vi "PingPongBRAMTop.vi"(5 "Memories":T3, 7 "ReverseLineRead?":bool, 8 "Input Valid":bool, 9 "Line Status In":T2, 11 "Data In":i16[](array[numeric])=[0, 0, 0, 0]) -> (0 "Output Valid":bool, 1 "Line Status Out":T2, 3 "Data Out":i16[](array[numeric]))   [LabVIEW 2014]
doc: "This VI ping pongs data between two Block RAM (memory)."
uses:
  Acquisition Engine/Acquisition Status.ctl
panel:
  # "Copyright 2014 Vidrio Technologies\nScanImage 5 software is licensed under the Apache License, Version 2.0 (the \"License\"); you may not use any files contained\nwithin the ScanImage 5 release except in compliance with the License. You may obtain a copy of the License at\n http://www.apache.org/licenses/LICENSE-2.0\nUnless required by applicable law or agreed to in writing, software distributed under the License is distributed on an\n\"AS IS\" BASIS, WITHOUT WARRANTIES OR CONDITIONS OF ANY KIND, either express or implied. See the License for the\n specific language governing permissions and limitations under the License."
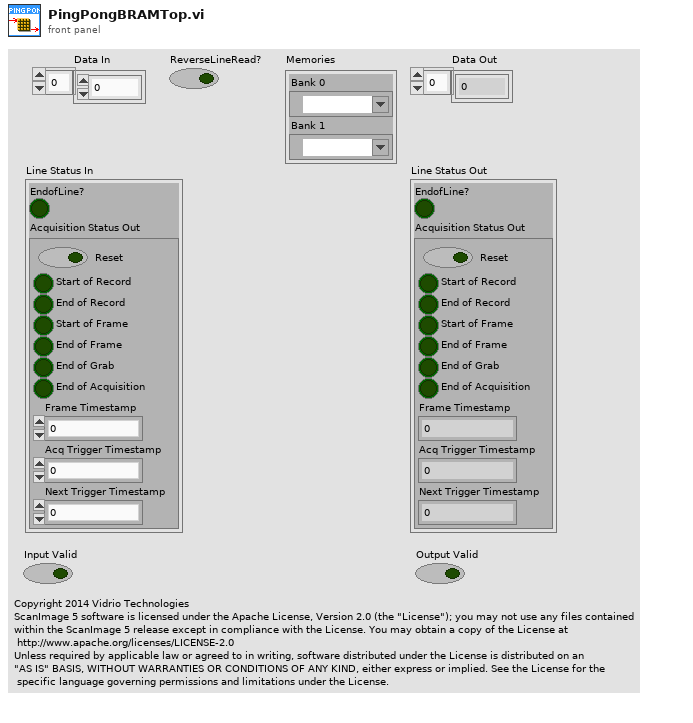
[diagram p1: front panel]
types:
  T1 = typedef "Acquisition Status.ctl" = cluster{"Reset":bool, "Start of Record":bool, "End of Record":bool, "Start of Frame":bool, "End of Frame":bool, "End of Grab":bool, "End of Acquisition":bool, "Frame Timestamp":u64, "Acq Trigger Timestamp":u64, "Next Trigger Timestamp":u64}
  T2 = cluster{"EndofLine?":bool, "Acquisition Status Out":T1}
  T3 = cluster{"Bank 0":refnum<k21>, "Bank 1":refnum<k21>}
  T4 = cluster{"Pixel Data":i16[], "Timestamps":cluster{"Frame Timestamp":u64, "Acq Trigger Timestamp":u64, "Next Trigger Timestamp":u64}}
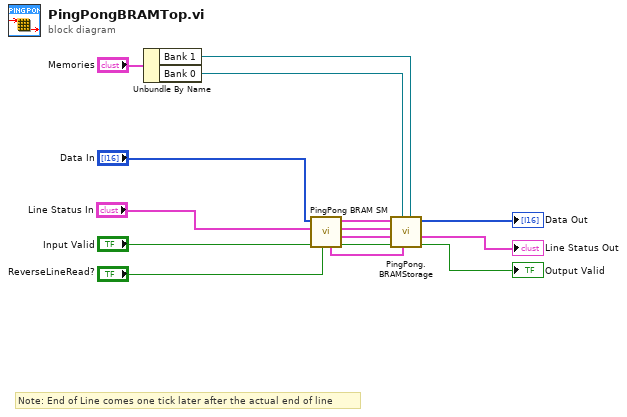
[diagram p0: block diagram]
diagram:
  # "Note: End of Line comes one tick later after the actual end of line"
  n1 = Unbundle By Name("Memories") -> ("Bank 1"=w5:refnum<k21>, "Bank 0"=w6:refnum<k21>)
  n2 = call "PingPong BRAM SM.vi"("Reverse Read?"="ReverseLineRead?", "Input Valid"="Input Valid", "Line Status In"="Line Status In", "Input"="Data In") -> ("BRAM Bank0 Write?"=w12:bool, "Read Info"=w13:cluster{"Read Address":u16, "Read Valid":bool}, "Write Info"=w14:cluster{"Write Address":u16, "Write Valid":bool}, "Frame Data Out"=w15:T4, "Line Status Out"=w4:T2)  [unwired: 3 in]
  n3 = call "PingPong.BRAMStorage.vi"("Bank 1"=w5, "Line Status In"=w4, "Bank 0"=w6, "BRAM Bank0 Write?"=w12, "Read Info"=w13, "Write Info"=w14, "Frame Data In"=w15) -> ("Output Valid"=→"Output Valid":bool, "Line Status Out"=→"Line Status Out":T2, "Data Out"=→"Data Out":i16[])  [unwired: 2 in]
